vi "XML Parse.vi"() -> ()   [LabVIEW 2016]
doc: "Reads an array of temperature data, including the max, min, and average temperature from an XML file created by the Write Data to XML File.vi example. The VI then unflattens this data to LabVIEW data and displays it on the front panel.\n\n<B>Temp Graph</B> displays the data after the VI collects all of the data"
uses:
  <vilib>/xml/Close Reference(Node).vi
  <vilib>/xml/NI_XML.lvlib
  <resource>/objmgr/DOMUserDefRef.rc
  <vilib>/httpClient/LabVIEWHTTPClient.lvlib
panel:
  out "number":i32
  out "name 2":string
  out "error out 2":errorcluster
  out "name":string
  out "error out":errorcluster
  # "Note: Write Data to XML File.vi must be run before executing this VI, as it writes the XML data file\nthat is read in this VI.  Select Help»Show Context Help and move the cursor over the VI icon \nfor more information."
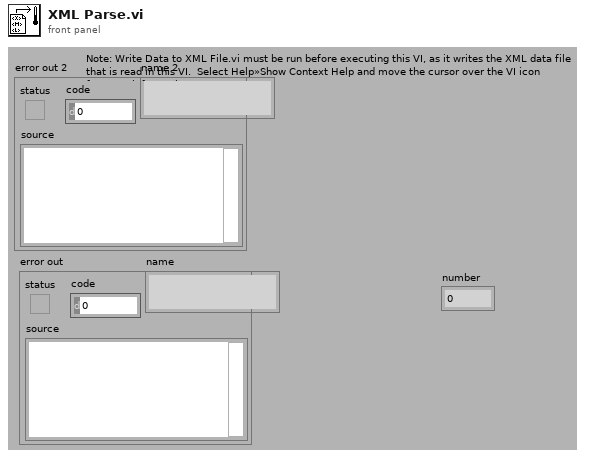
[diagram p1: front panel]
types:
  T1 = typedef "LabVIEWHTTPClient.lvlib/ClientHandle.ctl" = refnum<k1>
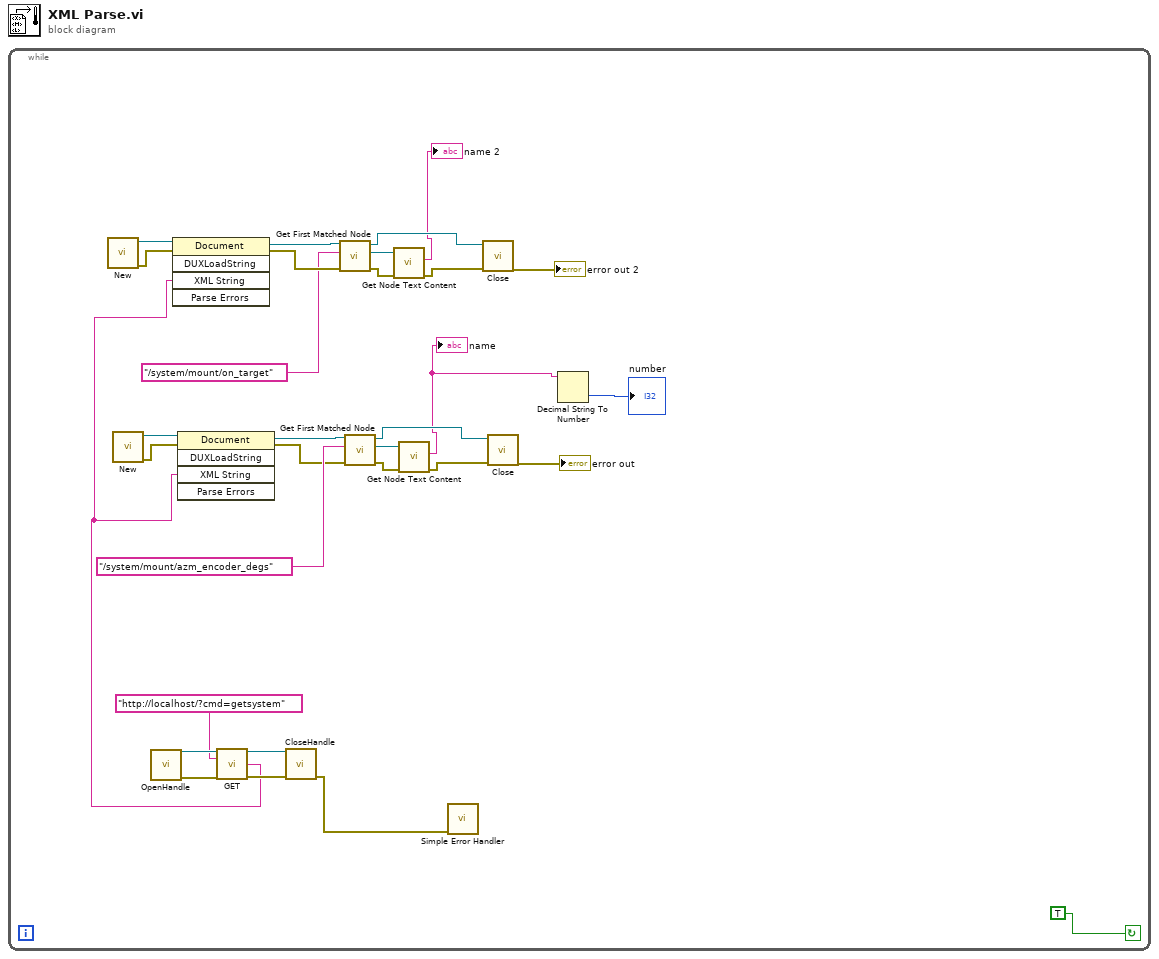
[diagram p0: block diagram]
diagram:
  n1 = while {
    stop <- TRUE continue-if-true
    n2 = call <vilib>:"New.vi"() -> ("error out"=w6:errorcluster, "DOM document out"=w5:refnum<k20>)  [unwired: 8 in]
    n3 = call <vilib>:"New.vi"() -> ("error out"=w30:errorcluster, "DOM document out"=w31:refnum<k20>)  [unwired: 8 in]
    n4 = call <vilib>:"OpenHandle.vi"() -> ("client handle out"=w24:T1, "error out"=w27:errorcluster)  [unwired: 14 in]
    n5 = call <vilib>:"GET.vi"("client handle"=w24, "url"="http://localhost/?cmd=getsystem" ("Webpage URL"), "error in (no error)"=w27) -> ("client handle out"=w25:T1, "body"=w4:string, "error out"=w26:errorcluster)  [unwired: 9 in, 1 out]
    n6 = invoke class="Document" method="DUXLoadString"(reference=w5, error in=w6, "XML String"=w4) -> (reference out=w9:refnum<k20>, error out=w8:errorcluster)  [unwired: 2 in, 3 out]
    n7 = invoke class="Document" method="DUXLoadString"(reference=w31, error in=w30, "XML String"=w4) -> (reference out=w21:refnum<k20>, error out=w28:errorcluster)  [unwired: 2 in, 3 out]
    n8 = call <vilib>:"CloseHandle.vi"("client handle"=w25, "error in (no error)"=w26) -> ("error out"=w23:errorcluster)  [unwired: 13 in]
    n9 = call <vilib>:"Get First Matched Node.vi"("error in (no error)"=w8, "XPath expression"="/system/mount/on_target", "node in"=w9) -> ("error out"=w11:errorcluster, "node result"=w12:refnum<k20>, "node out"=w14:refnum<k20>)  [unwired: 6 in]
    n10 = call <vilib>:"Get First Matched Node.vi"("error in (no error)"=w28, "XPath expression"="/system/mount/azm_encoder_degs", "node in"=w21) -> ("error out"=w19:errorcluster, "node result"=w18:refnum<k20>, "node out"=w17:refnum<k20>)  [unwired: 6 in]
    n11 = call <vilib>:"Get Node Text Content.vi"("error in (no error)"=w11, "node in"=w12) -> ("error out"=w15:errorcluster, "node text"=→"name 2":string)  [unwired: 7 in, 1 out]
    n12 = call <vilib>:"Get Node Text Content.vi"("error in (no error)"=w19, "node in"=w18) -> ("error out"=w16:errorcluster, "node text"=w2:string)  [unwired: 7 in, 1 out]
    "name" <- w2
    n13 = call <vilib>:"Simple Error Handler.vi"("error in (no error)"=w23) -> ()  [unwired: 4 in, 5 out]
    n14 = call-poly <vilib>:"Close.vi"("error in (no error)"=w15, "node"=w14) -> ("error out"=→"error out 2":errorcluster)  [unwired: 7 in]
    n15 = call-poly <vilib>:"Close.vi"("error in (no error)"=w16, "node"=w17) -> ("error out"=→"error out":errorcluster)  [unwired: 7 in]
    n16 = Decimal String To Number(string=w2) -> (number=→"number":i32)  [unwired: 2 in, 1 out]
  }
